vi "getState.vi"(5 "LabVIEW Web Service Request":refnum<class "Web Request.lvclass">) -> (4 "Response":string)   [LabVIEW 2024]
uses:
  <vilib>/wsapi/Web Request.lvclass
  Global.vi
panel:
  # "Use the Web Service Request input terminal to call the VIs on the Web Services palette. Do not remove it from the connector pane unless you don't need access to the palette."
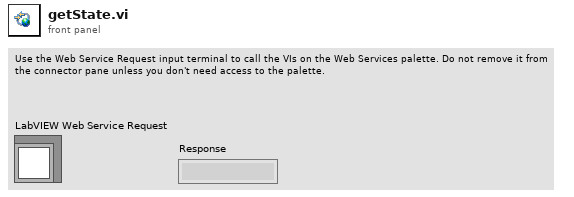
[diagram p1: front panel]
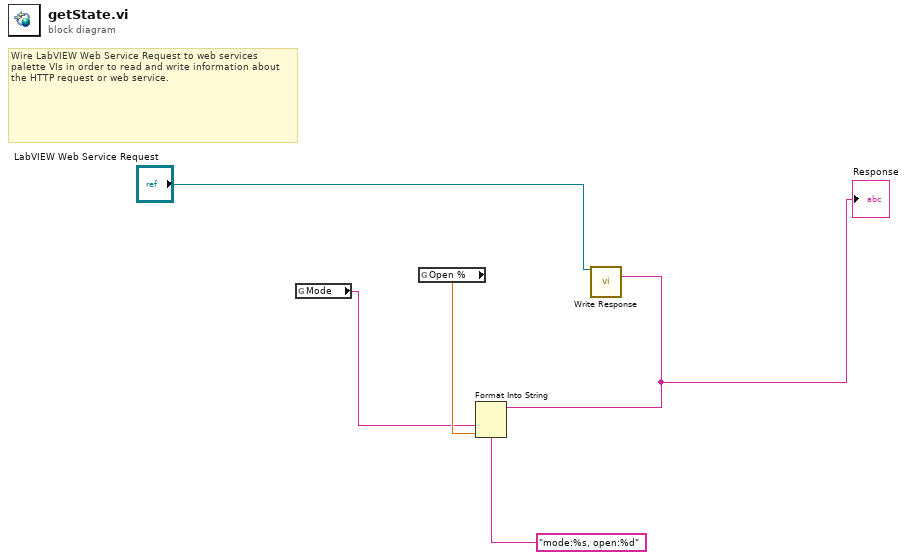
[diagram p0: block diagram]
diagram:
  # "Wire LabVIEW Web Service Request to web services palette VIs in order to read and write information about the HTTP request or web service."
  n1 = global read "Global.vi" "Mode"() -> (w2:string)
  n2 = global read "Global.vi" "Open %"() -> (w3:dbl)
  n3 = Format Into String(format string="mode:%s, open:%d", w2, w3) -> (resulting string=w1:string)  [unwired: 2 in, 1 out]
  "Response" <- w1
  n4 = call <vilib>:"Write Response.vi"("LabVIEW Web Service Request"="LabVIEW Web Service Request", "response string"=w1) -> ()  [unwired: 12 in, 2 out]
